vi "Actor Core.vi"(8 "error in":errorcluster, 11 "User Manager Model in":refnum<class "User Manager Model.lvclass">=refnum) -> (0 "error out":errorcluster, 3 "Actor out":refnum<class "Actor.lvclass">)   [LabVIEW 2017, in "User Manager Model.lvlib" / "User Manager Model.lvclass"]
doc: "(<B>Filename</B>: Actor Framework.lvlib:Actor.lvclass:Actor Core.vi)\n\nReceives messages to the actor, reacts to them, and initiates any error handling that may shut the actor down.\n\nDescendant classes may override this VI to append parallel tasks for the actor to complete while it handles messages. Overrides use the Call Parent Method node."
uses:
  User Manager Model.lvclass
  <vilib>/gpm_packages/@cs/mva-core/Source/IObserver/IObserver/IObserver.lvclass
  <vilib>/gpm_packages/@cs/mva-core/Source/SubscriptionPolicy/BasicSubscription/BasicSubscription.lvclass
  User Manager Model Messages/Login Msg/Login Msg.lvclass
  User Manager Model Messages/Logout Msg/Logout Msg.lvclass
  Type Definitions/Credentials.ctl
  Type Definitions/User Manager Application Types.lvlib
  User Manager Model Messages/Add User Msg/Add User Msg.lvclass
  User Manager Model Messages/Get All Users Msg/Get All Users Msg.lvclass
  User Manager Model Messages/Remove User Msg/Remove User Msg.lvclass
  Type Definitions/New User Information.ctl
  C:/CS Dev/LabVIEW Modules/composed-user-manager application/gpm_packages/@cs/mva-framework/Source/Framework/IObserver/IObserver/IObserver.lvclass
  User Manager Model Messages/Get User's Password Msg/Get User's Password Msg.lvclass
  User Manager Model Messages/Get User Attribute Msg/Get User Attribute Msg.lvclass
  Type Definitions/User Levels.ctl
  C:/Program Files/National Instruments/LabVIEW 2017/vi.lib/ActorFramework/Actor/Actor.lvclass
  C:/Program Files/National Instruments/LabVIEW 2017/vi.lib/gpm_packages/@cs/mva-core/Source/IMediator/ISubscriptionPolicy/ISubscriptionPolicy.lvclass
  C:/Program Files/National Instruments/LabVIEW 2017/vi.lib/gpm_packages/@cs/transport/Source/Concrete/ActorMessageTransport/Notification Msg/Notification Msg.lvclass
  C:/Program Files/National Instruments/LabVIEW 2017/vi.lib/gpm_packages/@cs/actor-framework-messages/Source/RoundTripMessage/RoundTripMessage.lvclass
  C:/Program Files/National Instruments/LabVIEW 2017/vi.lib/ActorFramework/Message/Message.lvclass
  <vilib>/ActorFramework/Actor/Actor.lvclass
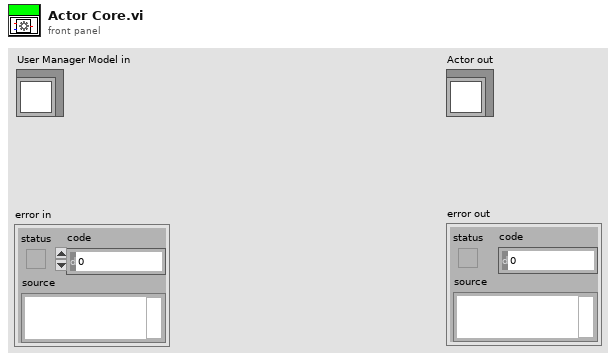
[diagram p1: front panel]
types:
  T1 = typedef "User Manager Application Types.lvlib/New User Information.ctl" = cluster{"User Info":T2, "User Level":T3}
  T2 = typedef "User Manager Application Types.lvlib/Credentials.ctl" = cluster{"Username":string, "Password":string}
  T3 = typedef "User Manager Application Types.lvlib/User Levels.ctl" = cluster{"Rank":i32, "Title":string}
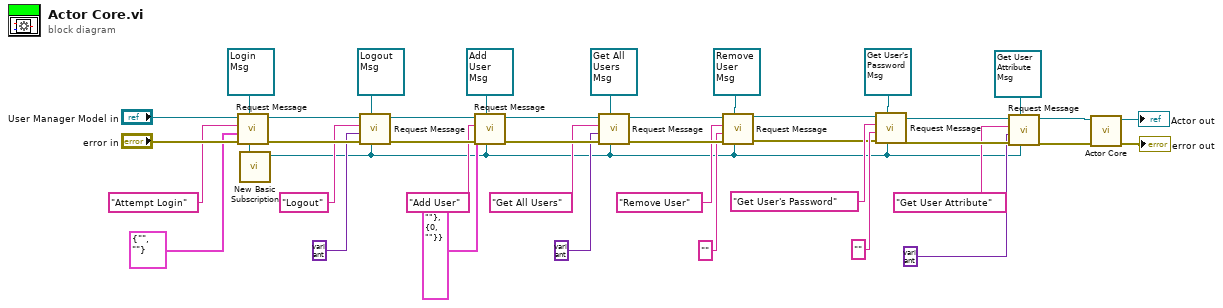
[diagram p0: block diagram]
diagram:
  n1 = call <vilib>:"New Basic Subscription.vi"() -> ("BasicSubscription Out"=w1:refnum<class "BasicSubscription.lvclass">)  [unwired: 11 in]
  n2 = call <vilib>:"Request Message.vi"("Configured SubscriptionPolicy"=w1, "Desired Notification Msg"=refnum<class "Login Msg.lvclass"> refnum ("User Manager Model.lvlib:Login Msg.lvclass"), "error in (no error)"="error in", "Data Type"=T2 {"Username"="", "Password"=""} ("User Credentials"), "Datum Name"="Attempt Login", "IObserver in"="User Manager Model in") -> ("error out"=w37:errorcluster, "IObserver out"=w38:refnum<class "IObserver.lvclass">)  [unwired: 3 in, 1 out]
  n3 = call <vilib>:"Request Message.vi"("Configured SubscriptionPolicy"=w1, "Desired Notification Msg"=refnum<class "Logout Msg.lvclass"> refnum ("User Manager Model.lvlib:Logout Msg.lvclass"), "error in (no error)"=w37, "Data Type"=variant ("element"), "Datum Name"="Logout", "IObserver in"=w38) -> ("error out"=w35:errorcluster, "IObserver out"=w36:refnum<class "IObserver.lvclass">)  [unwired: 3 in, 1 out]
  n4 = call <vilib>:"Request Message.vi"("Configured SubscriptionPolicy"=w1, "Desired Notification Msg"=refnum<class "Add User Msg.lvclass"> refnum ("User Manager Model.lvlib:Add User Msg.lvclass"), "error in (no error)"=w35, "Data Type"=T1 {"User Info"={"Username"="", "Password"=""}, "User Level"={"Rank"=0, "Title"=""}} ("New Uer Info"), "Datum Name"="Add User", "IObserver in"=w36) -> ("error out"=w33:errorcluster, "IObserver out"=w34:refnum<class "IObserver.lvclass">)  [unwired: 3 in, 1 out]
  n5 = call <vilib>:"Request Message.vi"("Configured SubscriptionPolicy"=w1, "Desired Notification Msg"=refnum<class "Get All Users Msg.lvclass"> refnum ("User Manager Model.lvlib:Get All Users Msg.lvclass"), "error in (no error)"=w33, "Data Type"=variant ("element"), "Datum Name"="Get All Users", "IObserver in"=w34) -> ("error out"=w31:errorcluster, "IObserver out"=w32:refnum<class "IObserver.lvclass">)  [unwired: 3 in, 1 out]
  n6 = call <vilib>:"Request Message.vi"("Configured SubscriptionPolicy"=w1, "Desired Notification Msg"=refnum<class "Remove User Msg.lvclass"> refnum ("User Manager Model.lvlib:Remove User Msg.lvclass"), "error in (no error)"=w31, "Data Type"="" ("Username"), "Datum Name"="Remove User", "IObserver in"=w32) -> ("error out"=w10:errorcluster, "IObserver out"=w11:refnum<class "IObserver.lvclass">)  [unwired: 3 in, 1 out]
  n7 = call <vilib>:"Request Message.vi"("Configured SubscriptionPolicy"=w1, "Desired Notification Msg"=refnum<class "Get User's Password Msg.lvclass"> refnum ("User Manager Model.lvlib:Get User's Password Msg.lvclass"), "error in (no error)"=w10, "Data Type"="" ("Username"), "Datum Name"="Get User's Password", "IObserver in"=w11) -> ("error out"=w7:errorcluster, "IObserver out"=w8:refnum<class "IObserver.lvclass">)  [unwired: 3 in, 1 out]
  n8 = call <vilib>:"Request Message.vi"("Configured SubscriptionPolicy"=w1, "Desired Notification Msg"=refnum<class "Get User Attribute Msg.lvclass"> refnum ("User Manager Model.lvlib:Get User Attribute Msg.lvclass"), "error in (no error)"=w7, "Data Type"=variant, "Datum Name"="Get User Attribute", "IObserver in"=w8) -> ("error out"=w3:errorcluster, "IObserver out"=w4:refnum<class "IObserver.lvclass">)  [unwired: 3 in, 1 out]
  n9 = call-parent "Actor Core.vi"("error in"=w3, "Actor in"=w4) -> ("error out"=→"error out":errorcluster, "Actor out"=→"Actor out":refnum<class "Actor.lvclass">)  [unwired: 8 in]
